vi "Handle Message.vi"(0 "Message Handler In":refnum<class "Message Handler.lvclass">, 7 "Message In":T1, 11 "Error In":errorcluster) -> (4 "Message Handler Out":refnum<class "Message Handler.lvclass">, 6 "CMD Out":string, 8 "Message Out":T1, 15 "Error Out":errorcluster)   [LabVIEW 2023, in "Message Handler.lvclass"]
uses:
  Message Handler.lvclass
  Interfaces/ICanCommunicate/Message.ctl
  Interfaces/ICanCommunicate/ICanCommunicate.lvclass
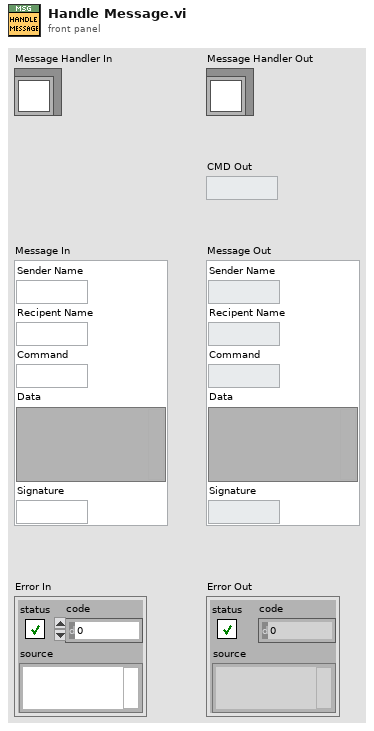
[diagram p1: front panel]
types:
  T1 = typedef "ICanCommunicate.lvclass/Message.ctl" = cluster{"Sender Name":string, "Recipent Name":string, "Command":string, "Data":variant, "Signature":string}
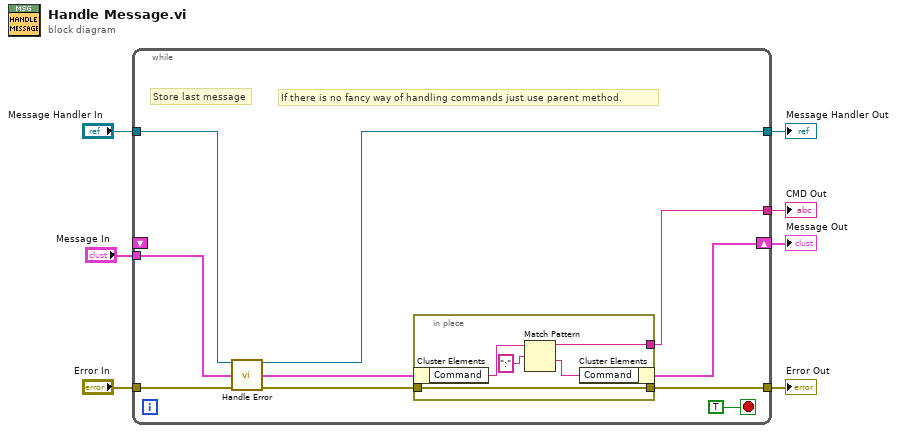
[diagram p0: block diagram]
diagram:
  n1 = while {
    shift-right: [w9] -> w3
    shift-left: _ -> [_]
    tunnel: "Error In" -> [w16]
    tunnel: [w11] -> w6
    tunnel: "Message Handler In" -> [w14]
    tunnel: [w13] -> w4
    tunnel: "Message In" -> [w15]
    tunnel: [w10] -> w1
    stop <- TRUE stop-if-true
    # "If there is no fancy way of handling commands just use parent method."
    # "Store last message"
    n2 = call-dynamic "Handle Error.vi"("Process In"=w14, "Message In"=w15, "Error In"=w16) -> ("Process Out"=w13:refnum<class "Message Handler.lvclass">, "Message Out"=w8:T1, "Error Out"=w12:errorcluster)  [unwired: 10 in]
    n3 = in-place {
      in-place-border: [w20] -> w10
      in-place-border: [w18] -> w11
      in-place-border: w12 -> [w18]
      n4 = in-place-cluster #1(w8) -> ("Command"=w21:string)
      n5 = Match Pattern(string=w21, regular expression=":") -> (before substring=w20:string, after substring=w19:string)  [unwired: 1 in, 2 out]
      n6 = in-place-cluster #1("Command"=w19) -> (w9:T1)
    }
  }
  "Error Out" <- w6
  "Message Handler Out" <- w4
  "Message Out" <- w3
  "CMD Out" <- w1
